vi "User Event Reference Handler.vi"(7 "Reference Action":T1, 8 "Error In":errorcluster, 10 "Event Registration Refnum In":refnum<event-registration>, 11 "User Event Refnum In":refnum<user-event>) -> (0 "Error Out":errorcluster, 2 "Event Registration Refnum Out":refnum<event-registration>, 3 "User Event Refnum Out":refnum<user-event>)   [LabVIEW 2017]
uses:
  Reference Action.ctl
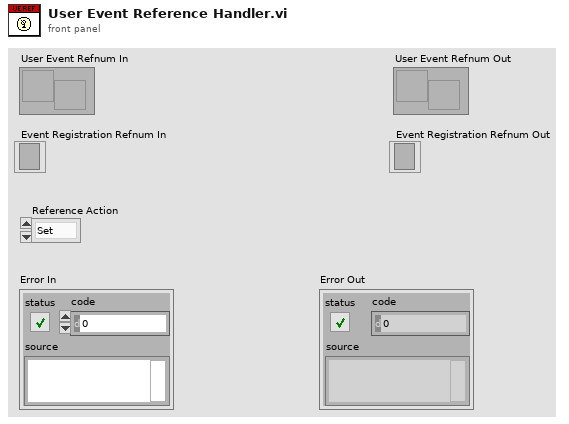
[diagram p1: front panel]
types:
  T1 = typedef "Reference Action.ctl" = enum16{"Set", "Get"}
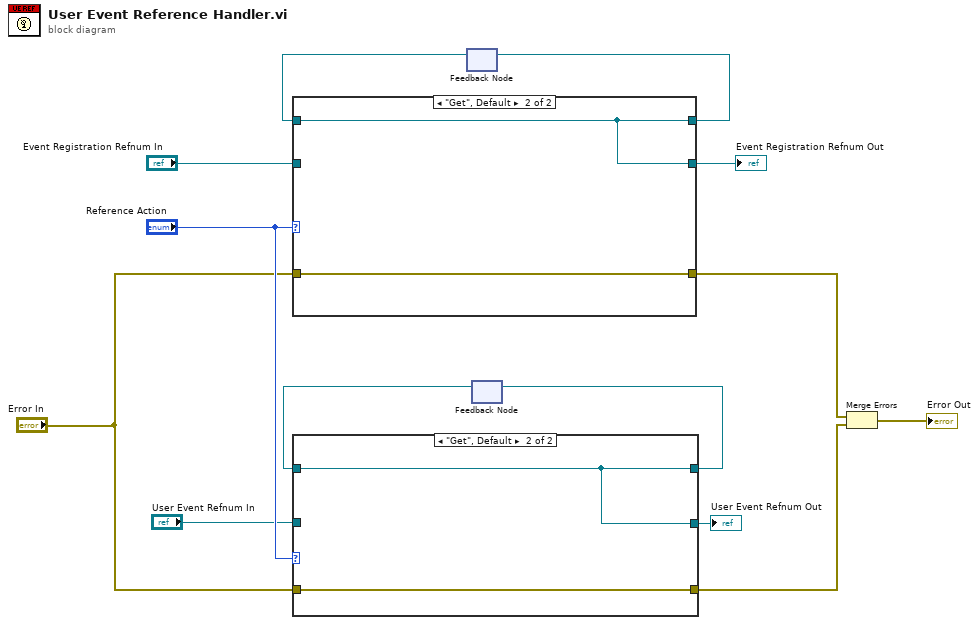
[diagram p0: block diagram]
diagram:
  n1 = feedback #1() -> (w12:refnum<event-registration>)  [unwired: 1 in]
  n2 = case shown="\"Get\", Default" "Reference Action" {
    tunnel: "Event Registration Refnum In" -> [w15 _]
    tunnel: [w15 w17] -> w3
    tunnel: [w15 w17] -> w13
    tunnel: w12 -> [_ w17]
    tunnel: [w14 w16] -> w7
    tunnel: "Error In" -> [w14 w16]
    frame "Set" {
    }
    frame "Get", Default {
    }
  }
  "Event Registration Refnum Out" <- w3
  n3 = feedback-in #1(w13) -> ()
  n4 = feedback #2() -> (w9:refnum<user-event>)  [unwired: 1 in]
  n5 = case shown="\"Get\", Default" "Reference Action" {
    tunnel: "User Event Refnum In" -> [w19 _]
    tunnel: [w19 w21] -> w1
    tunnel: [w19 w21] -> w10
    tunnel: w9 -> [_ w21]
    tunnel: "Error In" -> [w18 w20]
    tunnel: [w18 w20] -> w5
    frame "Set" {
    }
    frame "Get", Default {
    }
  }
  "User Event Refnum Out" <- w1
  n6 = feedback-in #2(w10) -> ()
  n7 = Merge Errors(w7, w5) -> (→"Error Out":errorcluster)
